vi "Initialise EEPROM.vi"() -> (3 "EEPROM":u8[](array[numeric]))   [LabVIEW 2021]
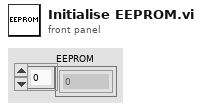
[diagram p1: front panel]
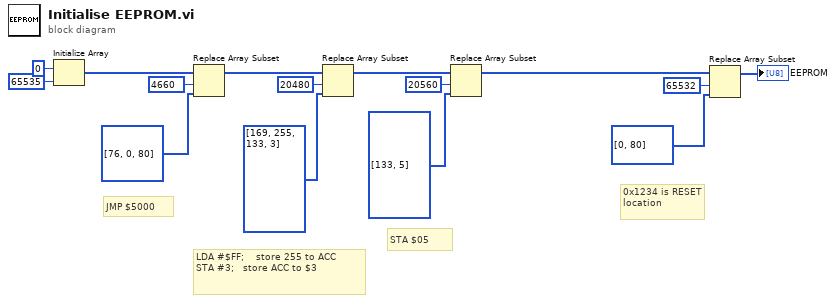
[diagram p0: block diagram]
diagram:
  # "STA $05"
  # "LDA #$FF;    store 255 to ACC\nSTA #3;   store ACC to $3"
  # "0x1234 is RESET location"
  # "JMP $5000"
  n1 = Initialize Array(u8 0 ("element"), 65535 ("dimension size")) -> (w10:u8[])
  n2 = Replace Array Subset(array=w10, new element=u8[] [76, 0, 80], index=u16 4660) -> (w7:u8[])
  n3 = Replace Array Subset(array=w7, new element=u8[] [169, 255, 133, 3], index=20480) -> (w3:u8[])
  n4 = Replace Array Subset(array=w3, new element=u8[] [133, 5], index=20560) -> (w1:u8[])
  n5 = Replace Array Subset(array=w1, new element=u8[] [0, 80], index=u16 65532) -> (→"EEPROM":u8[])
